vi "MODBUS Test.vi"() -> ()   [LabVIEW 2014]
uses:
  <vilib>/NI/Modbus Library/API/Wrapper/Create Serial Master.vi
  <vilib>/NI/Modbus Library/API/Master/Modbus Master.lvclass
  <vilib>/NI/Modbus Library/API/Wrapper/API Main.lvlib
panel:
  in  "number of inputs":u16=1
  in  "starting address":u16=65535
  in  "error in":errorcluster
  out "error out":errorcluster
  in  "Register to write 2":u16
  in  "coil to write":bool
  in  "Register to write":sgl
  in  "stop":bool
  out "*(type *) &x":sgl[](array[numeric])
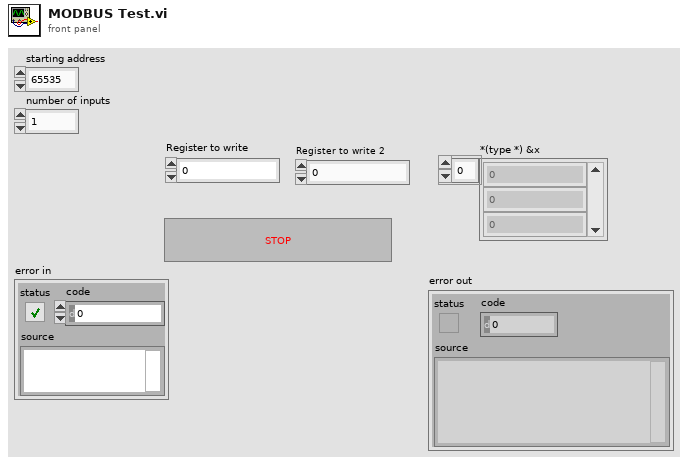
[diagram p1: front panel]
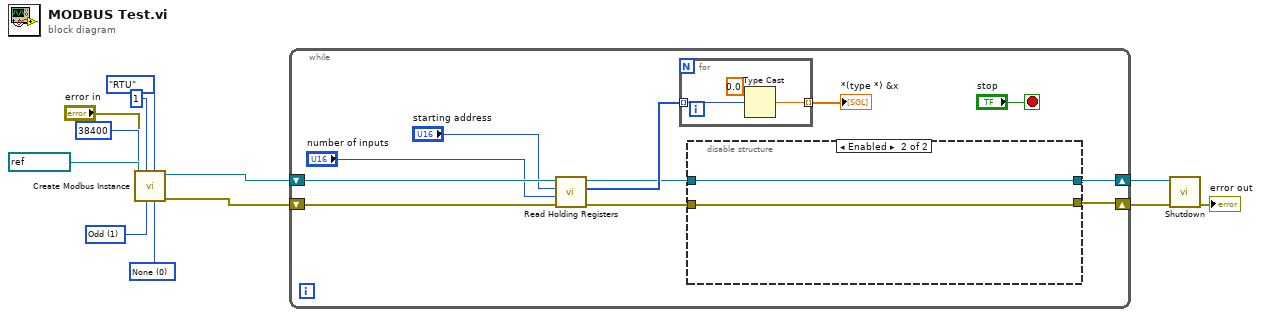
[diagram p0: block diagram]
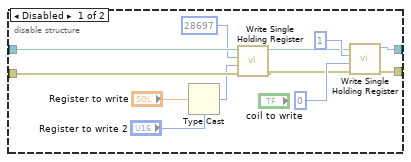
[diagram p2: hidden frame]
diagram:
  w2 = u16 1 items=["None", "Odd", "Even", "Mark", "Space"] ("parity (even)")
  w3 = u16 0 items=["None", "XON/XOFF", "RTS/CTS", "XON/XOFF & RTS/CTS", "DTR/DSR", "XON/XOFF & DTR/DSR"] ("flow control (none)")
  n1 = call-poly <vilib>:"Create Modbus Instance.vi"("flow control (none)"=w3, "serial type"=enum16{"RTU", "ASCII"}."RTU", "parity (even)"=w2, "unit ID"=u8 1, "error in"="error in", "baud rate"=u32 38400, "VISA resource name"=refnum<visa-resource-name> "COM4") -> ("error out"=w8:errorcluster, "serial master instance"=w9:refnum<class "Modbus Master.lvclass">)  [unwired: 3 in]
  n2 = while {
    shift-right: [w14] -> w12
    shift-left: w9 -> [w23]
    shift-right: [w13] -> w11
    shift-left: w8 -> [w22]
    stop <- "stop" stop-if-true
    n3 = call-dynamic "Read Holding Registers.vi"("error in"=w22, "number of inputs"="number of inputs", "starting address"="starting address", "Modbus master in"=w23) -> ("error out"=w15:errorcluster, "register values"=w19:u16[], "Modbus master out"=w16:refnum<class "Modbus Master.lvclass">)  [unwired: 5 in]
    n4 = for {
      tunnel: w19 -> [w40] mode=indexing
      tunnel: [w39] -> w18 mode=indexing
      n5 = Type Cast(type=sgl 0.0, x=w40) -> (*(type *) &x=w39:sgl)
    }
    "*(type *) &x" <- w18
    n6 = disable-structure shown="Enabled" {
      disable-tunnel: w16 -> [w35 w37]
      disable-tunnel: w15 -> [w34 w36]
      disable-tunnel: [w29 w37] -> w14
      disable-tunnel: [w28 w36] -> w13
      frame Disabled {
        n7 = Type Cast(type="Register to write 2", x="Register to write") -> (*(type *) &x=w30:u16)
        n8 = call-dynamic "Write Single Holding Register.vi"("error in"=w34, "register to write"=w30, "address"=u16 28697, "Modbus master in"=w35) -> ("error out"=w24:errorcluster, "Modbus master out"=w25:refnum<class "Modbus Master.lvclass">)  [unwired: 6 in]
        n9 = call-dynamic "Write Single Holding Register.vi"("error in"=w24, "register to write"=u16 0, "address"=u16 1, "Modbus master in"=w25) -> ("error out"=w28:errorcluster, "Modbus master out"=w29:refnum<class "Modbus Master.lvclass">)  [unwired: 6 in]
      }
      frame Enabled {
      }
    }
  }
  n10 = call-dynamic "Shutdown.vi"("error in"=w11, "Modbus master in"=w12) -> ("error out"=→"error out":errorcluster)  [unwired: 9 in]
